vi "10_2.vi"() -> ()   [LabVIEW 2018]
panel:
  out "Solution":ext
  in  "Input":string="77\n10\n143\n46\n79\n97\n54\n116\n60\n91\n80\n132\n20\n154\n53\n14\n103\n31\n65\n110\n43\n38\n47\n120\n112\n87\n24\n95\n33\n104\n73\n22\n66\n137\n21\n109\n118\n63\n55\n124\n146\n148\n84\n86\n147\n125\n23\n85\n117\n71\n48\n136\n151\n130\n83\n56\n140\n9\n49\n113\n131\n133\n74\n37\n127\n34\n32\n106\n1\n78\n11\n72\n40\n96\n17\n64\n92\n102\n123\n126\n90\n105\n57\n99\n27\n70\n98\n111\n30\n50\n67\n2\n155\n5\n119\n8\n39"
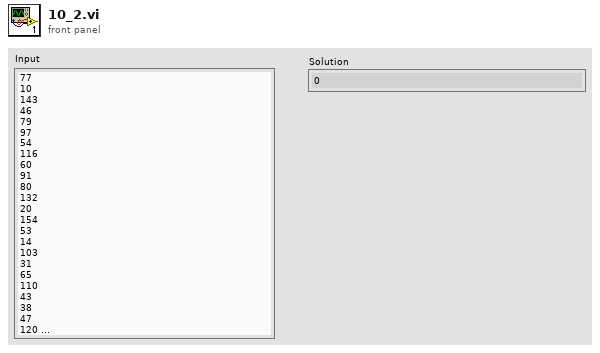
[diagram p1: front panel]
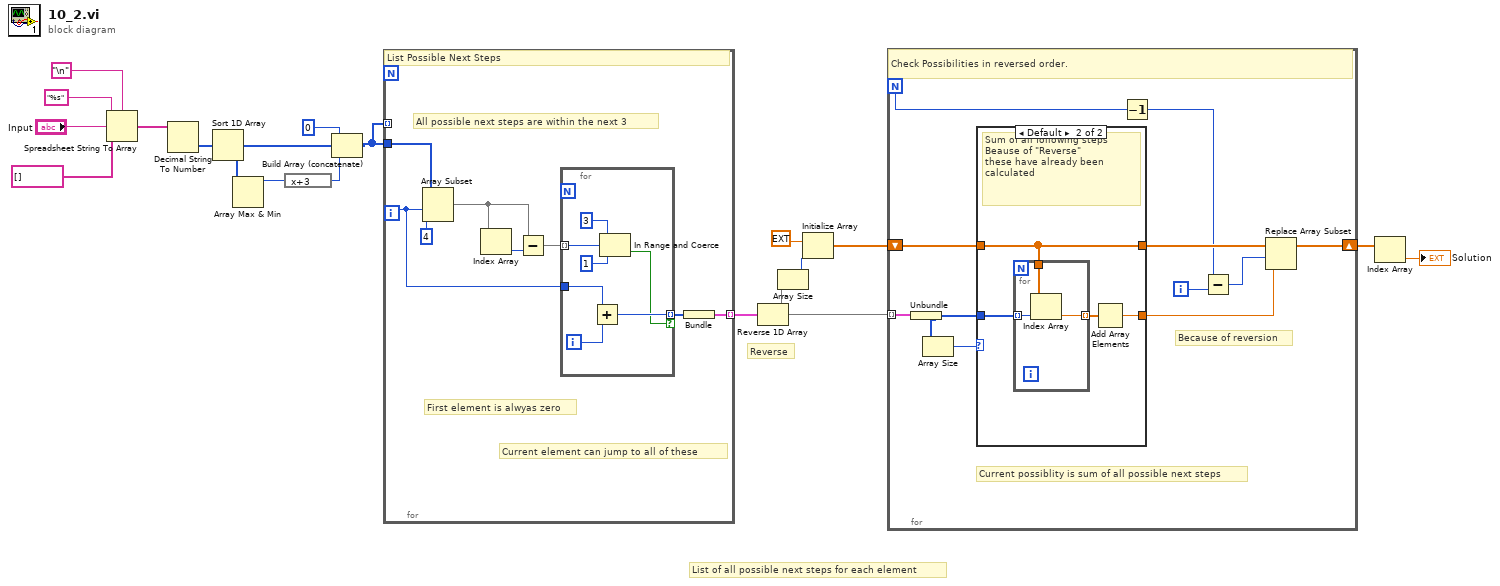
[diagram p0: block diagram]
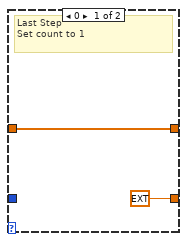
[diagram p2: hidden frame]
diagram:
  # "List of all possible next steps for each element"
  # "Reverse"
  n1 = Spreadsheet String To Array(delimiter (Tab)="\n", format string="%s", spreadsheet string="Input", array type (2D Dbl)=string[] []) -> (array=w14:string[])
  n2 = Decimal String To Number(string=w14) -> (number=w13:i32[])  [unwired: 2 in, 1 out]
  n3 = Sort 1D Array(array=w13) -> (sorted array=w11:i32[])
  n4 = Array Max & Min(array=w11) -> (max value=w12:i32)  [unwired: 3 out]
  n5 = expression code="x+3"(w12) -> (w9:i32)
  n6 = Build Array (concatenate)(0, w11, w9) -> (w8:i32[])
  n7 = for {
    tunnel: w8 -> [w24]
    tunnel: w8 -> [_] mode=indexing
    tunnel: [w19] -> w7 mode=indexing
    i -> [w21]
    # "Current element can jump to all of these"
    # "First element is alwyas zero"
    # "All possible next steps are within the next 3"
    # "List Possible Next Steps"
    n8 = Array Subset(array=w24, index=w21, length=4) -> (w22:i32[])
    n9 = Index Array(array=w22) -> (element=w26:i32)  [unwired: 1 in]
    n10 = Subtract(x=w22, y=w26) -> (x-y=w25:i32[])
    n11 = for {
      tunnel: w25 -> [w33] mode=indexing
      tunnel: w21 -> [w30]
      tunnel: [w28] -> w20 mode=indexing if=w27
      i -> [w29]
      n12 = Add(x=w30, y=w29) -> (x+y=w28:i32)
      n13 = In Range and Coerce(upper limit=3, x=w33, lower limit=1) -> (In Range?=w27:bool)  [unwired: 1 out]
    }
    n14 = Bundle(w20) -> (w19:cluster{i32[]})  [unwired: 1 in]
  }
  n15 = Reverse 1D Array(array=w7) -> (reversed array=w6:cluster{i32[]}[])
  n16 = Array Size(array=w6) -> (size(s)=w1:i32)
  n17 = Initialize Array(ext 0.0, w1) -> (w4:ext[])
  n18 = for {
    N -> [w38]
    tunnel: w6 -> [w44] mode=indexing
    shift-right: [w43] -> w3
    shift-left: w4 -> [w41]
    i -> [w36]
    # "Current possiblity is sum of all possible next steps"
    # "Because of reversion"
    # "Check Possibilities in reversed order."
    n19 = Unbundle(w44) -> (w34:i32[])
    n20 = Array Size(array=w34) -> (size(s)=w42:i32)
    n21 = case shown="Default" w42 {
      tunnel: w34 -> [_ w50]
      tunnel: w41 -> [w46 w47]
      tunnel: [w46 w47] -> w40
      tunnel: [ext 1.0 w48] -> w39
      frame 0 {
        # "Last Step\nSet count to 1"
      }
      frame Default {
        # "Sum of all following steps\nBeause of \"Reverse\"\nthese have already been calculated"
        n22 = for {
          tunnel: w50 -> [w53] mode=indexing
          tunnel: w47 -> [w52]
          tunnel: [w51] -> w49 mode=indexing
          n23 = Index Array(array=w52, index=w53) -> (element=w51:ext)
        }
        n24 = Add Array Elements(numeric array=w49) -> (sum=w48:ext)
      }
    }
    n25 = Decrement(x=w38) -> (x-1=w37:i32)
    n26 = Subtract(x=w37, y=w36) -> (x-y=w35:i32)
    n27 = Replace Array Subset(array=w40, new element=w39, index=w35) -> (w43:ext[])
  }
  n28 = Index Array(array=w3) -> (element=→"Solution":ext)  [unwired: 1 in]
